vi "Config Clipping.vi"(0 "VISA Resource Name":refnum<visa-resource-name>, 1 "Standard (0: IS-95A)":enum16{"IS-95A", "CDMA2000", "WCDMA"}(ring), 2 "Clipping Type  (0: |I + jQ|)":enum16{"|I + jQ|", "|I|, |Q|"}(ring), 3 "Clip |I| (100.0)":dbl=100.0, 4 "Clip |Q| (100.0)":dbl=100.0, 5 "error in (no error)":errorcluster {"code" format="%.0x"}, 6 "Clip |I + jQ| (100.0)":dbl=100.0, 7 "Clipping Filter  (0: PRE)":i16(ring) items=["PRE", "POST"]) -> (14 "VISA Resource Name Out":refnum<visa-resource-name>, 19 "error out":errorcluster {"code" format="%.0x"})   [LabVIEW 2012, in "Agilent ESG Series.lvlib"]
doc: "This VI configures clipping paramters."
uses:
  <instrlib>/Agilent ESG Series/Agilent ESG Series.lvlib
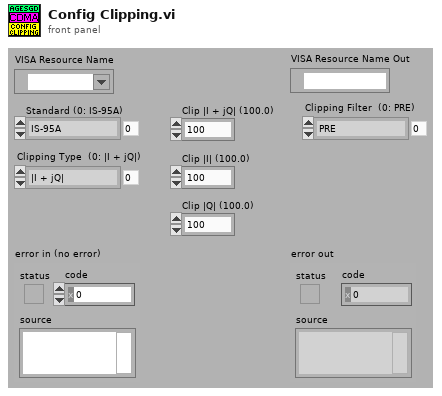
[diagram p1: front panel]
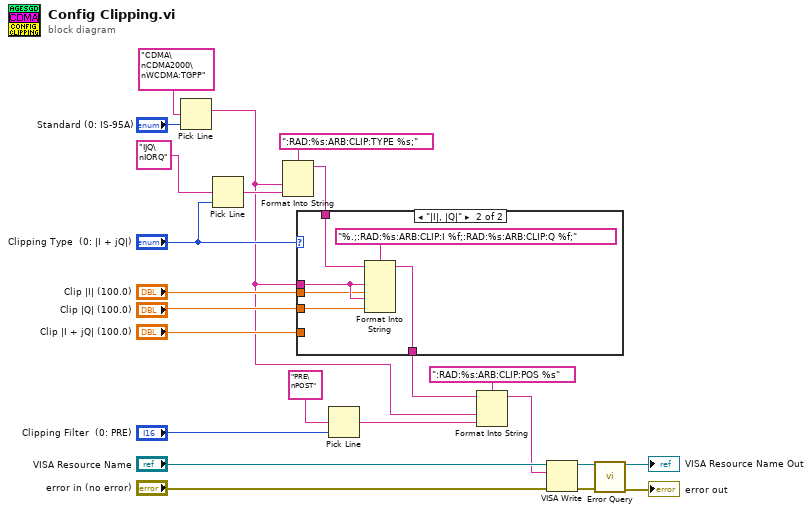
[diagram p0: block diagram]
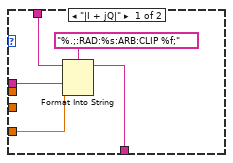
[diagram p2: hidden frame]
diagram:
  n1 = Pick Line(multi-line string="CDMA\nCDMA2000\nWCDMA:TGPP", line index="Standard (0: IS-95A)") -> (output string=w4:string)  [unwired: 1 in]
  n2 = Pick Line(multi-line string="IJQ\nIORQ", line index="Clipping Type  (0: |I + jQ|)") -> (output string=w14:string)  [unwired: 1 in]
  n3 = Format Into String(format string=":RAD:%s:ARB:CLIP:TYPE %s;", w4, w14) -> (resulting string=w11:string)  [unwired: 2 in, 1 out]
  n4 = case shown="\"|I|, |Q|\"" "Clipping Type  (0: |I + jQ|)" {
    tunnel: w11 -> [w27 w33]
    tunnel: w4 -> [w25 w32]
    tunnel: "Clip |I| (100.0)" -> [_ w31]
    tunnel: "Clip |Q| (100.0)" -> [_ w30]
    tunnel: "Clip |I + jQ| (100.0)" -> [w26 _]
    tunnel: [w24 w29] -> w3
    frame "|I + jQ|" {
      n5 = Format Into String(format string="%.;:RAD:%s:ARB:CLIP %f;", initial string=w27, w25, w26) -> (resulting string=w24:string)  [unwired: 1 in, 1 out]
    }
    frame "|I|, |Q|" {
      n6 = Format Into String(format string="%.;:RAD:%s:ARB:CLIP:I %f;:RAD:%s:ARB:CLIP:Q %f;", initial string=w33, w32, w31, w32, w30) -> (resulting string=w29:string)  [unwired: 1 in, 1 out]
    }
  }
  n7 = Pick Line(multi-line string="PRE\nPOST", line index="Clipping Filter  (0: PRE)") -> (output string=w5:string)  [unwired: 1 in]
  n8 = Format Into String(format string=":RAD:%s:ARB:CLIP:POS %s", initial string=w3, w4, w5) -> (resulting string=w1:string)  [unwired: 1 in, 1 out]
  n9 = VISA Write(VISA resource name="VISA Resource Name", write buffer=w1, error in (no error)="error in (no error)") -> (VISA resource name out=w19:refnum<visa-resource-name>, error out=w18:errorcluster)  [unwired: 1 out]
  n10 = call <instrlib>:"Error Query.vi"("VISA Resource Name"=w19, "error in (no error)"=w18) -> ("VISA Resource Name Out"=→"VISA Resource Name Out":refnum<visa-resource-name>, "error out"=→"error out":errorcluster)  [unwired: 10 in, 2 out]
